vi "reprGraphical.vi"(8 "error in (no error)":errorcluster, 9 "Image Descriptor":T1={"Upper-Left Corner Coordinates"={"UTM Zone"=0.0, "Hemisphere"=enum."North", "East"=0.0, "North"=0.0}, "Meters/Pixel"=42.294203} {"Upper-Left Corner Coordinates"."North" format="%#_10f"; "Upper-Left Corner Coordinates"."East" format="%#_8f"}, 10 "Image In":T3, 11 "StationKeeping in":refnum<class "StationKeeping.lvclass">) -> (0 "error out":errorcluster, 2 "Image Out":T3, 3 "StationKeeping out":refnum<class "StationKeeping.lvclass">)   [LabVIEW 2011, in "StationKeeping.lvclass"]
doc: "Draws the four corners of the station on the mission map. The Image Descriptor and the StationKeeping mission have relative positions to each other. Once this is determined, the point of interest symbols are drawn on the map at their locations on the map image, relative to the GPS coordinates of the map."
uses:
  StationKeeping.lvclass
  <vilib>/vision/Image Controls.llb/IMAQ Image.ctl
  0-OCU/0 Code/mission input/0-Image Descriptor.ctl
  2 Typedefs/UTM Location.ctl
  StationKeeping.lvclass/StationKeeping.ctl
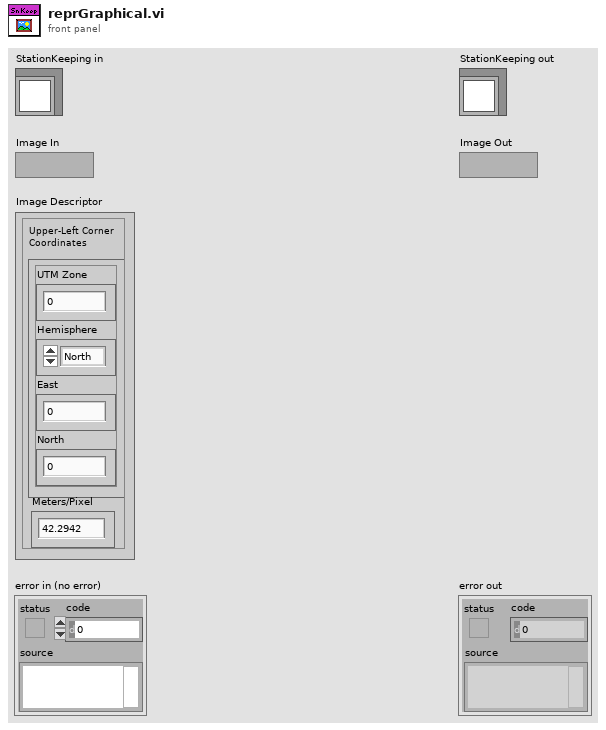
[diagram p1: front panel]
types:
  T1 = typedef "0-Image Descriptor.ctl" = cluster{"Upper-Left Corner Coordinates":T2, "Meters/Pixel":dbl}
  T2 = typedef "UTM Location.ctl" = cluster{"UTM Zone":dbl, "Hemisphere":enum16{"North", "South"}, "East":dbl, "North":dbl}
  T3 = typedef "IMAQ Image.ctl" = refnum<image>
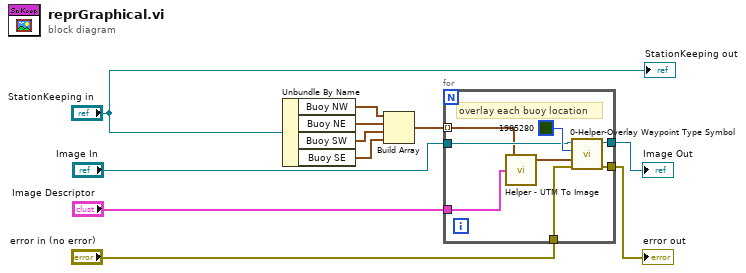
[diagram p0: block diagram]
diagram:
  n1 = Unbundle By Name("StationKeeping in") -> ("Buoy NW"=w10:T2, "Buoy NE"=w9:T2, "Buoy SW"=w8:T2, "Buoy SE"=w7:T2)
  n2 = Build Array(w10, w9, w8, w7) -> (w4:T2[])
  n3 = for {
    tunnel: [w17] -> w6
    tunnel: "Image In" -> [w16]
    tunnel: w4 -> [w15] mode=indexing
    tunnel: [w14] -> w3
    tunnel: "error in (no error)" -> [w13]
    tunnel: "Image Descriptor" -> [w12]
    # "overlay each buoy location"
    n4 = call "Helper - UTM To Image.vi"("Image Descriptor"=w12, "UTM Location"=w15) -> ("Pixel Coordinates"=w18:cluster{"X":i32, "Y":i32})  [unwired: 1 in, 2 out]
    n5 = call "0-Helper-Overlay Waypoint Type Symbol.vi"("error in"=w13, "Overlay Location"=w18, "Icon Color"=u32 1985280, "Image in"=w16) -> ("error out"=w14:errorcluster, "Image out"=w17:T3)  [unwired: 6 in]
  }
  "error out" <- w3
  "Image Out" <- w6
  "StationKeeping out" <- "StationKeeping in"
